vi "lab5-RTD.vi"() -> ()   [LabVIEW 2016]
uses:
  <vilib>/DAQmx/read.llb/DAQmx Read (Analog DBL 1Chan 1Samp).vi
  <vilib>/DAQmx/write.llb/DAQmx Write (Analog DBL 1Chan 1Samp).vi
  <vilib>/DAQmx/miscellaneous.llb/DAQmx Fill In Error Info.vi
panel:
  in  "task/channels in 2":refnum<k21>
  out "LED Voltage":i32
  out "Alarm(LED)":bool
  in  "Slide":dbl(slide) scale=0.0..100.0 scale format="%#.3g"
  out "Thermometer":dbl(slide) min=-25.0 max=125.0 scale=-25.0..125.0
  out "T":dbl
  in  "stop":bool
  out "Waveform Chart":dbl(graph)
  out "Vo":dbl format="%0.2f"
  in  "task/channels in":refnum<k21>
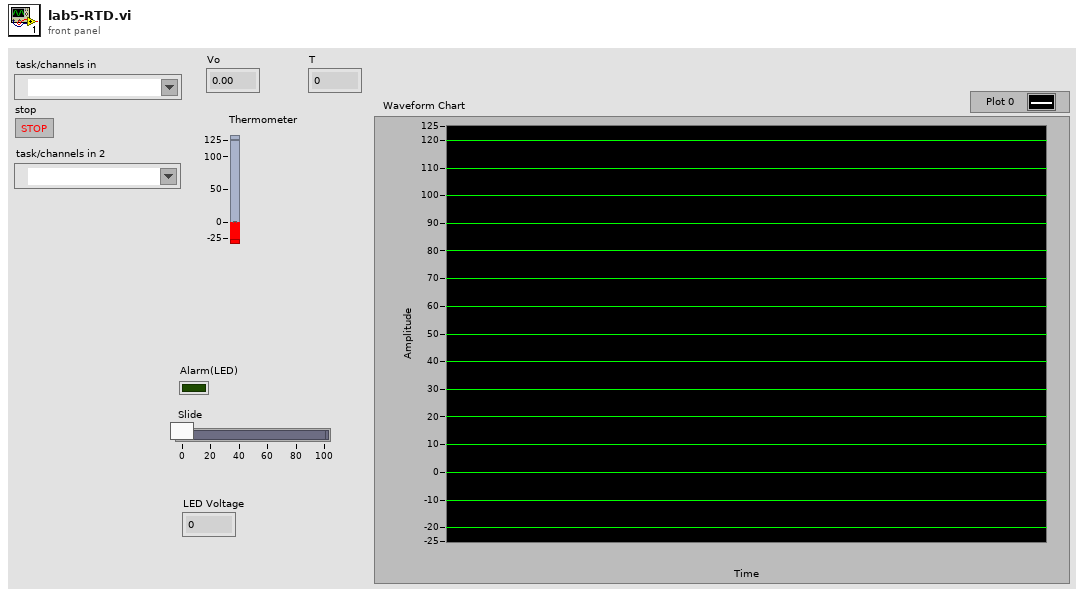
[diagram p1: front panel]
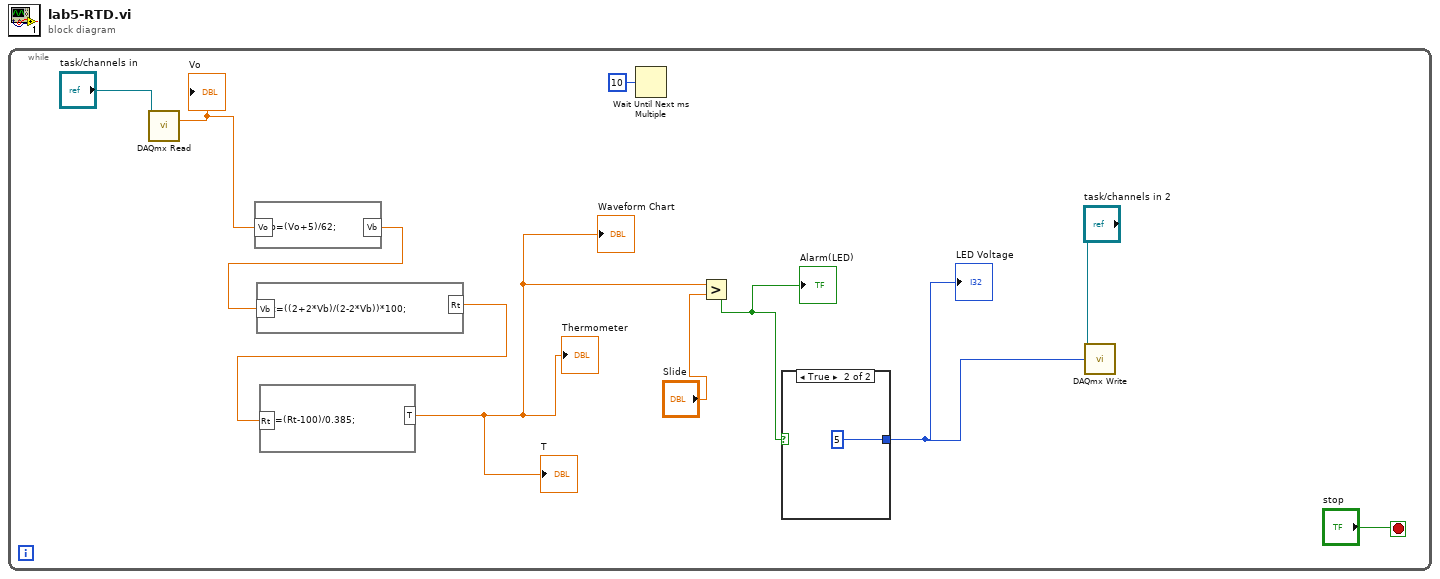
[diagram p0: block diagram]
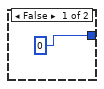
[diagram p2: hidden frame]
diagram:
  n1 = while {
    stop <- "stop" stop-if-true
    n2 = call-poly <vilib>:"DAQmx Read.vi"("task/channels in"="task/channels in") -> ("data"=w8:dbl)  [unwired: 12 in, 2 out]
    "Vo" <- w8
    n3 = formula code="Vb=(Vo+5)/62;"("Vo"=w8) -> ("Vb"=w7:dbl)
    n4 = formula code="Rt=((2+2*Vb)/(2-2*Vb))*100;"("Vb"=w7) -> ("Rt"=w6:dbl)
    n5 = formula code="T=(Rt-100)/0.385;"("Rt"=w6) -> ("T"=w5:dbl)
    "Waveform Chart" <- w5
    "T" <- w5
    "Thermometer" <- w5
    n6 = Wait Until Next ms Multiple(millisecond multiple=u32 10) -> ()  [unwired: 1 out]
    n7 = Greater?(x=w5, y="Slide") -> (0:w3:bool)
    "Alarm(LED)" <- w3
    n8 = case shown="True" w3 {
      tunnel: [0 5] -> w2
      frame False {
      }
      frame True {
      }
    }
    "LED Voltage" <- w2
    n9 = call-poly <vilib>:"DAQmx Write.vi"("task/channels in"="task/channels in 2", "data"=w2) -> ()  [unwired: 11 in, 3 out]
  }
